vi "getChamber.vi"(8 "error in (no error)":errorcluster, 11 "Instrument.Cryostat in":refnum<class "Instrument.Cryostat.lvclass">) -> (0 "error out":errorcluster, 2 "Status":string, 3 "Instrument.Cryostat out":refnum<class "Instrument.Cryostat.lvclass">)   [LabVIEW 2019, in "Instrument.Cryostat.lvclass"]
uses:
  Instrument.Cryostat.lvclass
  Instrument/Instrument.lvclass
  ae6c52b8-d0aa-4de2-ae58-6501a35f44e4.vi
  C:/Users/patrick/Documents/GitHub/Instrument-Framework/lvsrc/Instrument/Instrument.lvclass
  C:/Program Files (x86)/National Instruments/LabVIEW 2019/vi.lib/JKI/JKI SMO/SMO/SMO.lvclass
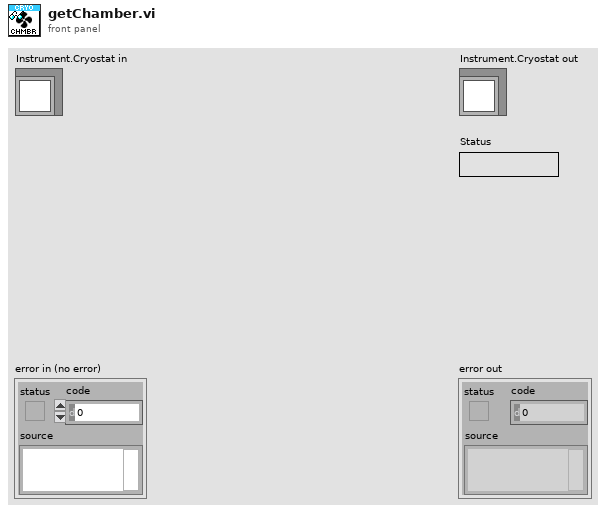
[diagram p1: front panel]
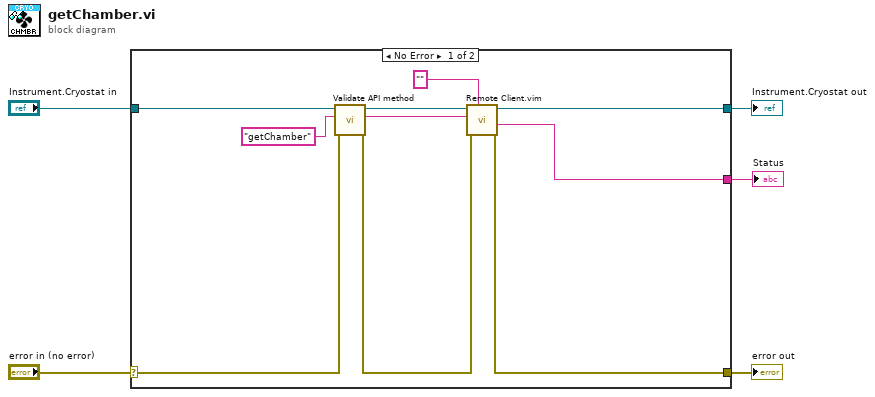
[diagram p0: block diagram]
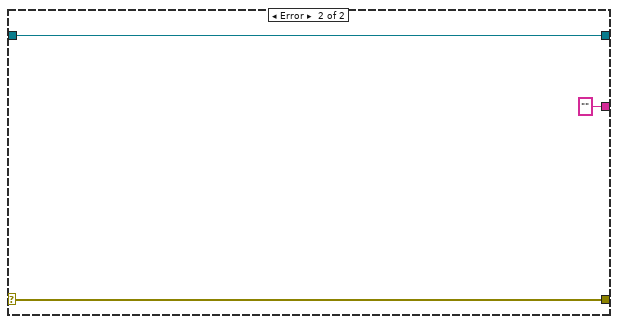
[diagram p2: hidden frame]
diagram:
  n1 = case shown="No Error" "error in (no error)" {
    selector: "error in (no error)" -> [w7 w18]
    tunnel: [w8 w18] -> w4
    tunnel: [w10 w17] -> w2
    tunnel: "Instrument.Cryostat in" -> [w11 w17]
    tunnel: [w9 "" ("Data out")] -> w1
    frame No Error {
      n2 = call "Validate API method.vi"("error in (no error)"=w7, "command in"="getChamber" ("error message (\"\")"), "Instrument in"=w11) -> ("error out"=w6:errorcluster, "command out"=w14:string, "Instrument out"=w13:refnum<class "Instrument.Cryostat.lvclass">)  [unwired: 6 in]
      n3 = call "Remote Client.vim"("Data Out type"="", "error in (no error)"=w6, "method"=w14, "Instrument in"=w13) -> ("error out"=w8:errorcluster, "Data out"=w9:string, "Instrument out"=w10:refnum<class "Instrument.Cryostat.lvclass">)  [unwired: 4 in, 1 out]
    }
    frame Error {
    }
  }
  "error out" <- w4
  "Instrument.Cryostat out" <- w2
  "Status" <- w1
